vi "Ini key read (DBL).vi"(7 "Section name":string, 8 "error in (no error)":errorcluster, 10 "Parameter names & setup":T2, 11 "Ini file refnum in":T1) -> (0 "error out":errorcluster, 2 "Value read/used":dbl[](array[numeric]), 3 "Ini file refnum out":T1)   [LabVIEW 2013]
uses:
  Typedefs/Ini file interface (DBL).ctl
  <vilib>/Utility/config.llb/Config Data RefNum.ctl
  <vilib>/Utility/config.llb/Read Key (Double).vi
  <vilib>/Utility/config.llb/Write Key (Double).vi
  <vilib>/Utility/config.llb/NI_LVConfig.lvlib
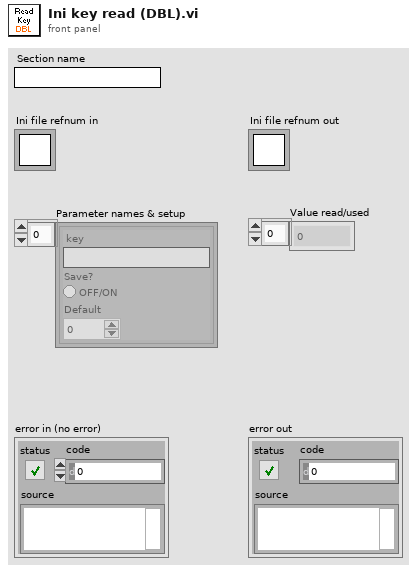
[diagram p1: front panel]
types:
  T1 = typedef "NI_LVConfig.lvlib/Config Data RefNum.ctl" = refnum<k1>
  T2 = typedef "Ini file interface (DBL).ctl" = cluster{"key":string, "Save?":bool, "Default":dbl}[]
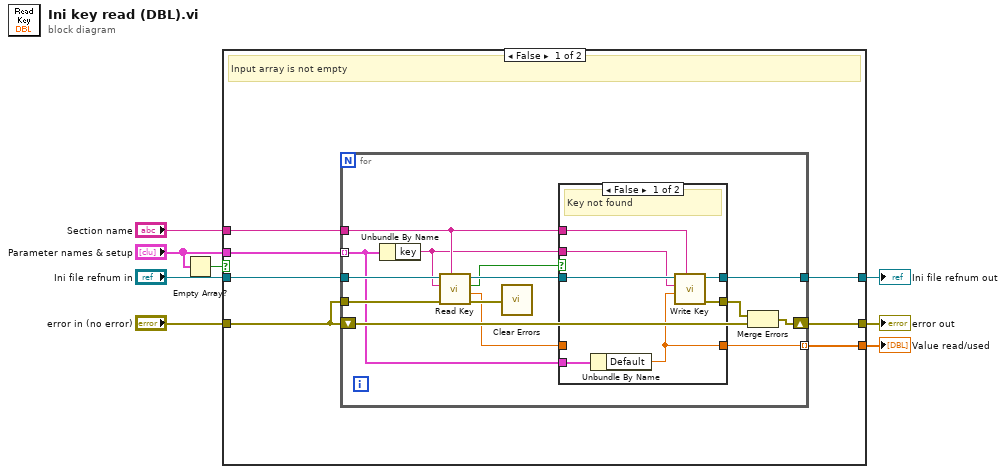
[diagram p0: block diagram]
diagram:
  n1 = Empty Array?(array="Parameter names & setup") -> (empty?=w1:bool)
  n2 = case shown="False" w1 {
    tunnel: "Section name" -> [w9 _]
    tunnel: "Parameter names & setup" -> [w15 _]
    tunnel: [w14 _] -> w7
    tunnel: "error in (no error)" -> [w10 w39]
    tunnel: [w13 w39] -> w5
    tunnel: [w12 w40] -> w4
    tunnel: "Ini file refnum in" -> [w11 w40]
    frame False {
      # "Input array is not empty"
      n3 = for {
        tunnel: w9 -> [w22]
        tunnel: w11 -> [w29]
        tunnel: w10 -> [w28]
        tunnel: [w25] -> w12
        shift-right: [w27] -> w13
        shift-left: w10 -> [w26]
        tunnel: w15 -> [w23] mode=indexing
        tunnel: [w24] -> w14 mode=indexing
        n4 = Unbundle By Name(w23) -> ("key"=w16:string)
        n5 = call-poly <vilib>:"Read Key.vi"("section"=w22, "error in (no error)"=w28, "key"=w16, "refnum"=w29) -> ("error out"=w21:errorcluster, "value"=w17:dbl, "found?"=w18:bool, "refnum out"=w20:T1)  [unwired: 4 in]
        n6 = call <vilib>:"Clear Errors.vi"("error in (no error)"=w21) -> ()  [unwired: 6 in, 1 out]
        n7 = case shown="False" w18 {
          tunnel: w20 -> [w36 w38]
          tunnel: [w35 w38] -> w25
          tunnel: [w34 _] -> w19
          tunnel: w22 -> [w33 _]
          tunnel: w16 -> [w32 _]
          tunnel: w17 -> [_ w37]
          tunnel: [w30 w37] -> w24
          tunnel: w23 -> [w31 _]
          frame False {
            # "Key not found"
            n8 = Unbundle By Name(w31) -> ("Default"=w30:dbl)
            n9 = call-poly <vilib>:"Write Key.vi"("section"=w33, "value"=w30, "key"=w32, "refnum"=w36) -> ("error out"=w34:errorcluster, "refnum out"=w35:T1)  [unwired: 5 in, 1 out]
          }
          frame True {
            # "Key found"
          }
        }
        n10 = Merge Errors(w19, w26) -> (w27:errorcluster)
      }
    }
    frame True {
      # "Input array is empty"
    }
  }
  "Value read/used" <- w7
  "error out" <- w5
  "Ini file refnum out" <- w4
